vi "niDAQmx Stop Task.vi"(0 "task in":refnum<class "Session Factory.lvclass">, 11 "error in":errorcluster) -> (4 "task out":refnum<class "Session Factory.lvclass">, 15 "error out":errorcluster)   [LabVIEW 2021, in "Session Management niDAQmx.lvlib" / "Session Factory.lvclass"]
doc: "Stops the task and returns it to the state the task was in before the DAQmx Start Task VI ran or the DAQmx Write VI ran with the <B>autostart</B> input set to TRUE."
uses:
  Session Factory.lvclass
  Sessions/niDAQmx/NI DAQmx Client/RPC Messages/nidaqmx_grpc_StopTaskRequest.ctl
  Sessions/niDAQmx/NI DAQmx Client/RPC Messages/nidevice_grpc_Session.ctl
  Sessions/niDAQmx/NI DAQmx Client/RPC Messages/nidevice_grpc_Session_session/nidevice_grpc_Session_session.lvclass
  Session Factory.lvclass/Session Factory.ctl
  Sessions/niDAQmx/NI DAQmx Client/NI_DAQmx_client.lvlib
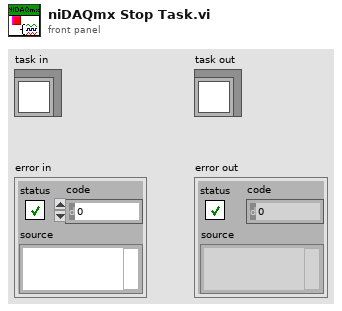
[diagram p1: front panel]
types:
  T1 = typedef "NI_DAQmx_client.lvlib/nidaqmx_grpc_StopTaskRequest.ctl" = cluster{"task":T2}
  T2 = typedef "NI_DAQmx_client.lvlib/nidevice_grpc_Session.ctl" = cluster{"nidevice_grpc_Session_session":refnum<class "nidevice_grpc_Session_session.lvclass">}
  T3 = typedef "grpc-lvsupport-release.lvlib/grpcId.ctl" = u64
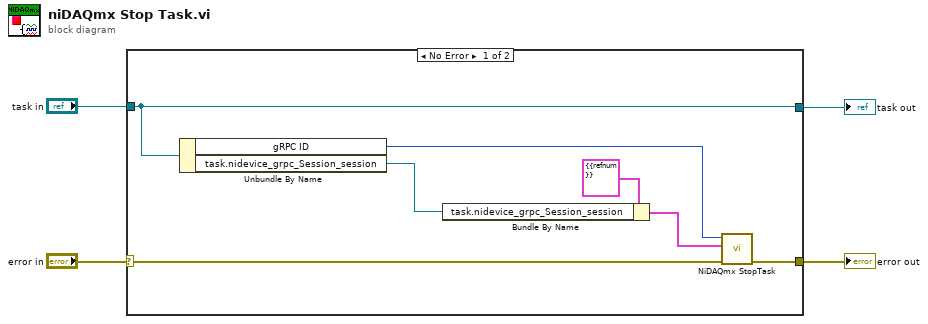
[diagram p0: block diagram]
diagram:
  n1 = case shown="No Error" "error in" {
    selector: "error in" -> [w10 w13]
    tunnel: [w9 w13] -> w3
    tunnel: "task in" -> [w11 w12]
    tunnel: [w11 w12] -> w1
    frame No Error {
      n2 = Unbundle By Name(w11) -> ("gRPC ID"=w8:T3, "task.nidevice_grpc_Session_session"=w5:refnum<class "nidevice_grpc_Session_session.lvclass">)
      n3 = Bundle By Name(cluster=T1 {"task"={"nidevice_grpc_Session_session"=refnum}} ("Request Data"), "task.nidevice_grpc_Session_session"=w5) -> (w6:T1)
      n4 = call "NiDAQmx StopTask.vi"("error in"=w10, "Request Data"=w6, "gRPC ID"=w8) -> ("error out"=w9:errorcluster)  [unwired: 6 in, 2 out]
    }
    frame Error {
    }
  }
  "error out" <- w3
  "task out" <- w1
